vi "PositionVoltage Setter.vi"(0 "DeviceReference":T1, 1 "Slot":i32, 3 "Update Frequency (Hz)":dbl=100.0, 5 "Position":dbl, 7 "EnableFOC":bool=TRUE, 9 "FeedForward":dbl) -> (4 "DeviceReference Out":T1)   [LabVIEW 2020]
doc: "Request PID to target position with duty-cycle feed forward.\nThis control mode will set the motor's position setpoint to the position specified by the user. In addition, it will apply an additional voltage as an arbitrary feed-forward value."
uses:
  DeviceReference.ctl
  <userlib>/CTRE_PhoenixTools/CTRE_PhoenixTools.lvlib
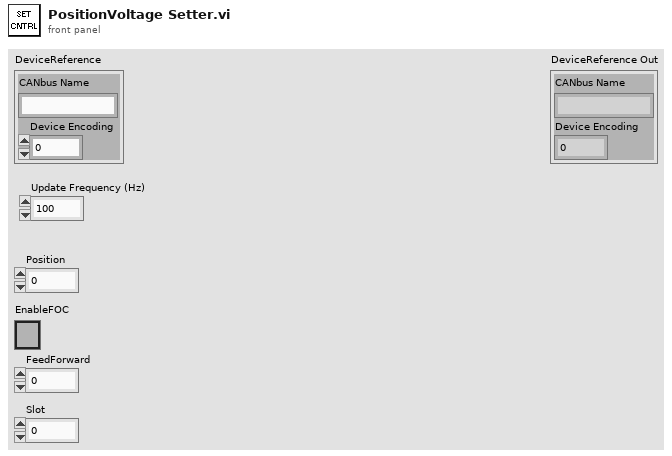
[diagram p1: front panel]
types:
  T1 = typedef "DeviceReference.ctl" = cluster{"CANbus Name":string, "Device Encoding":u32}
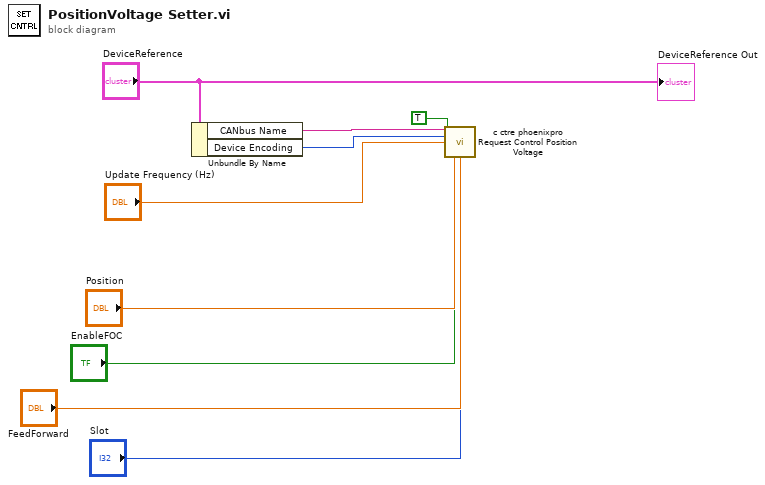
[diagram p0: block diagram]
diagram:
  n1 = Unbundle By Name("DeviceReference") -> ("CANbus Name"=w8:string, "Device Encoding"=w7:u32)
  n2 = call <userlib>:"c ctre phoenixpro Request Control Position Voltage.vi"("canbus"=w8, "Position"="Position", "FeedForward"="FeedForward", "ecuEncoding"=w7, "updateTime"="Update Frequency (Hz)", "cancelOtherRequests"=TRUE, "EnableFOC"="EnableFOC", "Slot"="Slot") -> ()  [unwired: 6 in, 2 out]
  "DeviceReference Out" <- "DeviceReference"
